vi "Release.vi"(8 "Error In":errorcluster, 11 "Timer Handle":T1) -> (0 "Error Out":errorcluster, 2 "Total Time(s)":dbl)   [LabVIEW 2016, in "Timer Session.lvclass"]
doc: "Releases an obtained reference to the timer."
uses:
  Timer Session.lvclass
  Typedefs/Session Handle.ctl
  Timer Session.lvclass/Timer Session.ctl
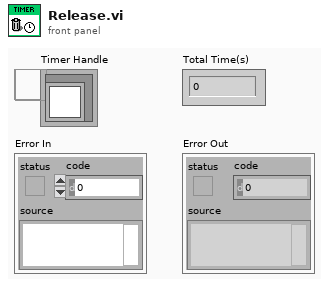
[diagram p1: front panel]
types:
  T1 = typedef "Timer Session.lvclass/Session Handle.ctl" = refnum<data-value>
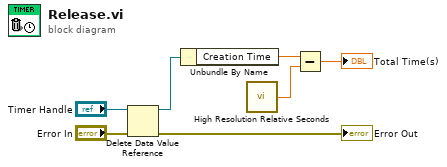
[diagram p0: block diagram]
diagram:
  n1 = Delete Data Value Reference(data value reference="Timer Handle", error in="Error In") -> (data value=w1:refnum<class "Timer Session.lvclass">, error out=→"Error Out":errorcluster)
  n2 = Unbundle By Name(w1) -> ("Creation Time"=w6:dbl)
  n3 = call <vilib>:"High Resolution Relative Seconds.vi"() -> ("relative seconds"=w7:dbl)
  n4 = Subtract(x=w6, y=w7) -> (x-y=→"Total Time(s)":dbl)
